vi "Event Handler.vi"(0 "uService Template in":refnum<class "DAQ Manager.lvclass">, 5 "Event type":T1=enum."Message", 7 "Item Name":string, 9 "Data":variant, 11 "error in (no error)":errorcluster) -> (4 "uService Template out":refnum<class "DAQ Manager.lvclass">, 15 "error out":errorcluster)   [LabVIEW 2020, in "DAQ Manager.lvlib" / "DAQ Manager.lvclass"]
doc: "This VI is the event handler of the uService: every time an event is triggered to the uService, this VI is called.\nNote: here you can access the Actor/Class data, but it will be the one coming out from Init. You cannot modify the values.\nThree different events are supported:\nI) Button Pressed: get called on a GUI button pressed. Item Name is the name (label) of the button, Data is empty.\nII) Shared Variable Updated: get called when a SV you subscribed to is updated. Item Name is the name of the SV, and Data is the value (note: you need to convert it to the proper type).\nIII) Message: get called every time a user event is generated using Send Message to Event Handler. The values of Item Name and Data are the one given to the Send Message to Event Handler.\nIV) Ready to launch?: this frame get called every time a new Run is initiated. Each uService is responsible of performing a self check before giving back the green light for the Run to start."
uses:
  DAQ Manager.lvclass
  C:/Users/marco/Documents/GitHub_Lab/TALOS/talos/Father of all uServices/Father of all uServices/Father of all uServices.lvclass
  Father of all uServices/Father of all uServices/Event Handler Items.ctl
  Ancestor/Ancestor/Ancestor.lvclass/Ancestor.ctl
  DAQ Manager Consumer Case Selector.ctl
  Father of all uServices/Father of all uServices Messages/Consumer Msg/Consumer Msg.lvclass/Consumer Msg.ctl
  Interfaces/DAQ Control/Metadata.ctl
  FGV/Error Memory/Get Error Description.vi
  Support VIs/Get PC name.vi
  Ancestor/Ancestor/Read ID.vi
  Support VIs/Get Class Name.vi
  <vilib>/Utility/error.llb/Clear Errors.vi
  Father of all uServices/Father of all uServices Messages/Consumer Msg/Send Consumer.vi
  FGV/Error Memory/Error Memory Core.vi
  <vilib>/AdvancedString/Delimited String to 1D String Array.vi
  Support VIs/Circus Root Path.vi
  FGV/Error Memory/Error Crt Lvl checker.vi
  FGV/Error Memory/Error Memory Core.vi/40c8088d-b597-4017-91af-faa98e00292e.vi
  FGV/Error Memory/Error Memory Core.vi/d4a3ab98-063c-4e44-b43d-fbdcfe6c2be2.vi
  Father of all uServices/Father of all uServices/Father of all uServices.lvclass
  C:/Users/marco/Documents/GitHub_Lab/TALOS/builds/Actor Framework PPL/Actor Framework.lvlibp/1abvi3w/vi.lib/ActorFramework/Actor/Actor.lvclass
  Support VIs/Global Memory.vi
  <vilib>/Utility/LVClass/Get LV Class Name.vi
  Support VIs/Is in Packed Library.vi
  Support VIs/TALOS Root path.vi
  Support VIs/Read CSV worksheet.vi
  Support VIs/Global Constants.vi
  <vilib>/Utility/error.llb/General Error Handler.vi
  builds/Actor Framework PPL/Actor Framework.lvlibp/1abvi3w/vi.lib/ActorFramework/Actor/Read Self Enqueuer.vi
  <userlib>/_OpenG.lib/lvdata/lvdata.llb/Get Strings from Enum__ogtk.vi
  builds/Actor Framework PPL/Actor Framework.lvlibp/1abvi3w/vi.lib/ActorFramework/Message Enqueuer/Enqueue.vi
  Support VIs/Error Log.vi
  Ancestor/Ancestor/Ancestor.lvclass
  <vilib>/Comparison/Equal/Equal Functor/Equal Functor.lvclass
  Father of all uServices/Father of all uServices Messages/Consumer Msg/Consumer Msg.lvclass
  Interfaces/DAQ Control/DAQ Control.lvclass
  TALOS.lvlib
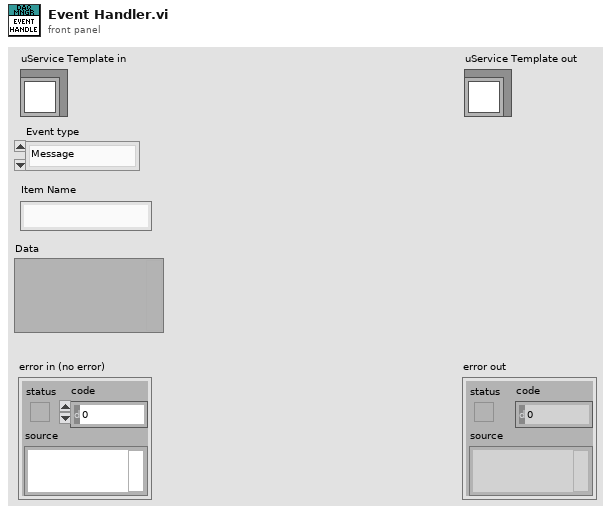
[diagram p1: front panel]
types:
  T1 = typedef "TALOS.lvlib/Father of all uServices.lvlib/Father of all uServices.lvclass/Event Handler Items.ctl" = enum16{"Button Pressed", "Shared Variable Updated", "Message", "Ready to launch?", "Safe Mode", "Start RUN", "Stop RUN"}
  T2 = typedef "DAQ Manager.lvlib/DAQ Manager.lvclass/DAQ Manager Consumer Case Selector.ctl" = enum16{"Start Run", "Get Run Status", "Stop Run", "Send metadata to DAQ", "Test send DAQ"}
  T3 = typedef "TALOS.lvlib/Interfaces.lvlib/DAQ Control.lvclass/Metadata.ctl" = cluster{"Key":string, "Value":string}
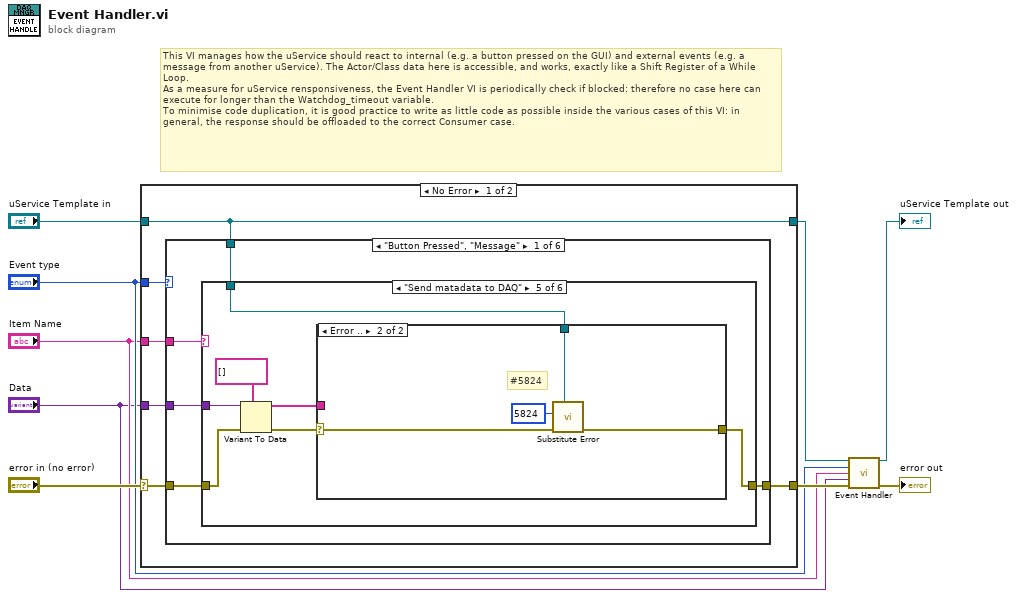
[diagram p0: block diagram]
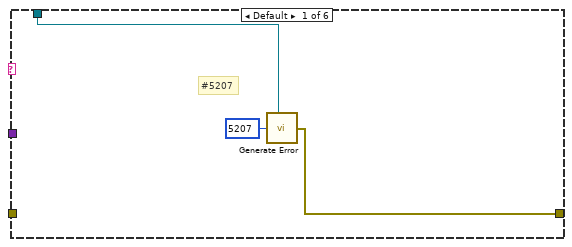
[diagram p2: hidden frame]
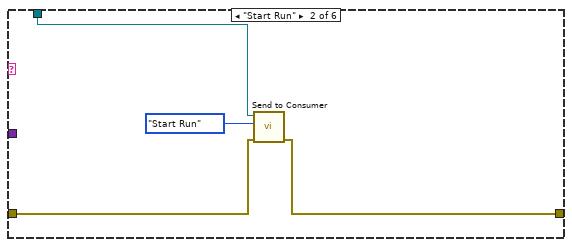
[diagram p3: hidden frame]
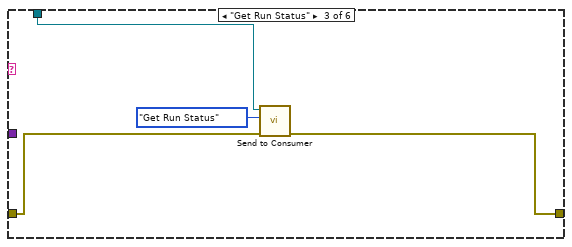
[diagram p4: hidden frame]
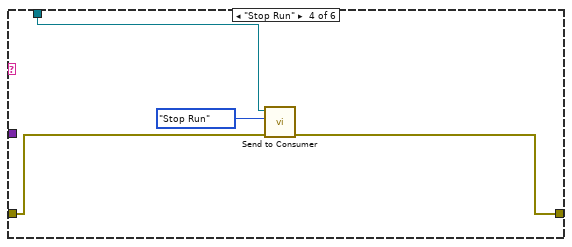
[diagram p5: hidden frame]
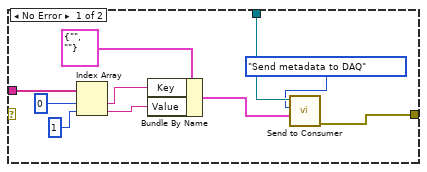
[diagram p6: hidden frame]
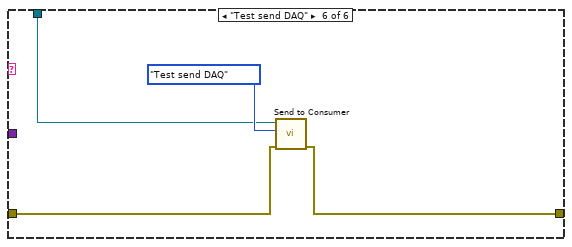
[diagram p7: hidden frame]
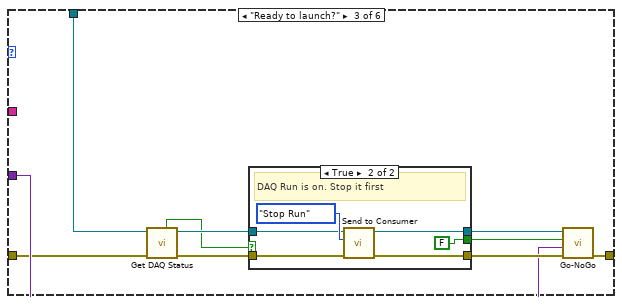
[diagram p9: hidden frame]
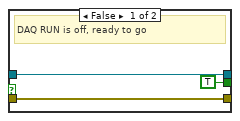
[diagram p10: hidden frame]
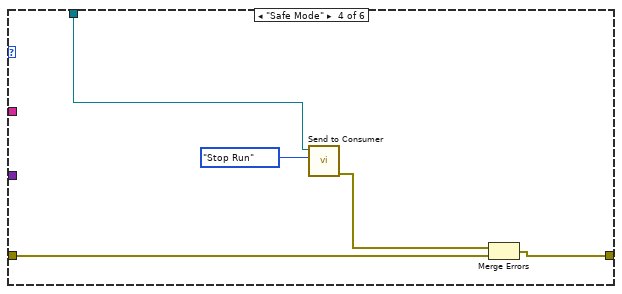
[diagram p11: hidden frame]
diagram:
  # "This VI manages how the uService should react to internal (e.g. a button pressed on the GUI) and external events (e.g. a message from another uService). The Actor/Class data here is accessible, and works, exactly like a Shift Register of a While Loop. \nAs a measure for uService rensponsiveness, the Event Handler VI is periodically check if blocked: therefore no case here can execute for longer than the Watchdog_timeout variable. \nTo minimise code duplication, it is good practice to write as little code as possible inside the various cases of this VI: in general, the response should be offloaded to the correct Consumer case."
  n1 = case shown="No Error" "error in (no error)" {
    selector: "error in (no error)" -> [w13 w89]
    tunnel: [w14 w89] -> w9
    tunnel: [w12 w88] -> w6
    tunnel: "uService Template in" -> [w12 w88]
    tunnel: "Event type" -> [w15 _]
    tunnel: "Item Name" -> [w11 _]
    tunnel: "Data" -> [w10 _]
    frame No Error {
      n2 = case shown="\"Button Pressed\", \"Message\"" w15 {
        tunnel: [w20 w61 w71 w83 w86 w87] -> w14
        tunnel: w13 -> [w17 w61 w62 w85 w86 w87]
        tunnel: w11 -> [w18 _ _ _ _ _]
        tunnel: w12 -> [w19 _ w65 w81 _ _]
        tunnel: w10 -> [w16 _ w68 _ _ _]
        frame "Button Pressed", "Message" {
          n3 = case shown="\"Send matadata to DAQ\"" w18 {
            tunnel: w17 -> [_ w27 w30 w34 w37 w59]
            tunnel: [w21 w26 w29 w33 w36 w58] -> w20
            tunnel: w19 -> [w22 w24 w28 w32 w39 w57]
            tunnel: w16 -> [_ _ _ _ w38 _]
            frame Default {
              # "#5207"
              n4 = call "Generate Error.vi"("Class"=w22, "Error Code"=5207) -> ("error out"=w21:errorcluster)  [unwired: 5 in]
            }
            frame "Start Run" {
              n5 = call "Send to Consumer.vi"("error in (no error)"=w27, "Case ID"=DAQ_Manager_Consumer_Case_Selector."Start Run" ("Consumer Case Selector"), "uService Template in"=w24) -> ("error out"=w26:errorcluster)  [unwired: 7 in, 1 out]
            }
            frame "Get Run Status" {
              n6 = call "Send to Consumer.vi"("error in (no error)"=w30, "Case ID"=DAQ_Manager_Consumer_Case_Selector."Get Run Status" ("Consumer Case Selector"), "uService Template in"=w28) -> ("error out"=w29:errorcluster)  [unwired: 7 in, 1 out]
            }
            frame "Stop Run" {
              n7 = call "Send to Consumer.vi"("error in (no error)"=w34, "Case ID"=DAQ_Manager_Consumer_Case_Selector."Stop Run" ("Consumer Case Selector"), "uService Template in"=w32) -> ("error out"=w33:errorcluster)  [unwired: 7 in, 1 out]
            }
            frame "Send matadata to DAQ" {
              n8 = Variant To Data(error in=w37, type=string[] [], Variant=w38) -> (data=w40:string[], error out=w41:errorcluster)
              n9 = case shown="Error .." w41 {
                selector: w41 -> [_ w56]
                tunnel: w39 -> [w52 w54]
                tunnel: [w51 w53] -> w36
                tunnel: w40 -> [w50 _]
                frame No Error {
                  n10 = Index Array(array=w50, index #1=0 ("index"), index #2=1 ("index")) -> (element #1=w46:string, element #2=w45:string)
                  n11 = Bundle By Name(cluster=T3 {"Key"="", "Value"=""}, "Key"=w46, "Value"=w45) -> (w44:T3)
                  n12 = call "Send to Consumer.vi"("Data"=w44, "Case ID"=DAQ_Manager_Consumer_Case_Selector."Send metadata to DAQ" ("Consumer Case Selector"), "uService Template in"=w52) -> ("error out"=w51:errorcluster)  [unwired: 7 in, 1 out]
                }
                frame Error {
                  # "#5824"
                  n13 = call "Substitute Error.vi"("LabVIEW Object"=w54, "error in (no error)"=w56, "Error Code"=5824) -> ("error out"=w53:errorcluster)  [unwired: 8 in]
                }
              }
            }
            frame "Test send DAQ" {
              n14 = call "Send to Consumer.vi"("error in (no error)"=w59, "Case ID"=DAQ_Manager_Consumer_Case_Selector."Test send DAQ" ("Consumer Case Selector"), "uService Template in"=w57) -> ("error out"=w58:errorcluster)  [unwired: 7 in, 1 out]
            }
          }
        }
        frame "Shared Variable Updated" {
        }
        frame "Ready to launch?" {
          n15 = call-dynamic "Get DAQ Status.vi"("error in (no error)"=w62, "DAQ Manager in"=w65) -> ("error out"=w63:errorcluster, "DAQ Manager out"=w66:refnum<class "DAQ Manager.lvclass">, "Run Active?"=w64:bool)  [unwired: 4 in, 3 out]
          n16 = case shown="True" w64 {
            tunnel: [TRUE ("Go?") FALSE ("Go?")] -> w69
            tunnel: w66 -> [w72 w75]
            tunnel: w63 -> [w73 w79]
            tunnel: [w73 w78] -> w70
            tunnel: [w72 w76] -> w67
            frame False {
              # "DAQ RUN is off, ready to go"
            }
            frame True {
              # "DAQ Run is on. Stop it first"
              n17 = call "Send to Consumer.vi"("error in (no error)"=w79, "Case ID"=DAQ_Manager_Consumer_Case_Selector."Stop Run" ("Consumer Case Selector"), "uService Template in"=w75) -> ("error out"=w78:errorcluster, "uService Template out"=w76:refnum<class "DAQ Manager.lvclass">)  [unwired: 7 in]
            }
          }
          n18 = call-dynamic "Go-NoGo.vi"("error in (no error)"=w70, "Go-NoGo Data"=w68, "Go?"=w69, "Father of all uServices in"=w67) -> ("error out"=w71:errorcluster)  [unwired: 6 in, 1 out]
        }
        frame "Safe Mode" {
          n19 = call "Send to Consumer.vi"("Case ID"=DAQ_Manager_Consumer_Case_Selector."Stop Run" ("Consumer Case Selector"), "uService Template in"=w81) -> ("error out"=w82:errorcluster)  [unwired: 8 in, 1 out]
          n20 = Merge Errors(w82, w85) -> (w83:errorcluster)
        }
        frame "Start RUN" {
        }
        frame "Stop RUN" {
        }
      }
    }
    frame Error {
    }
  }
  n21 = call-parent "Event Handler.vi"("uService Template in"=w6, "Event type"="Event type", "Item Name"="Item Name", "Data"="Data", "error in (no error)"=w9) -> ("uService Template out"=→"uService Template out":refnum<class "DAQ Manager.lvclass">, "error out"=→"error out":errorcluster)  [unwired: 9 in]
